vi "modbus-to-real.vi"(8 "error in (no error)":errorcluster, 11 "object in":refnum<class "Pressure-Transducer.lvclass">) -> (0 "error out":errorcluster, 3 "object out":refnum<class "Pressure-Transducer.lvclass">)   [LabVIEW 2021, in "Pressure-Transducer.lvclass"]
doc: "Uses adam formula to convert sensors to real No"
uses:
  Pressure-Transducer.lvclass
panel:
  # "Conversion for 4 to 20mA  and 0 to 10Vdc\ntransducer for the adam 4018+\n\nOutput the 4mA been subtracted."
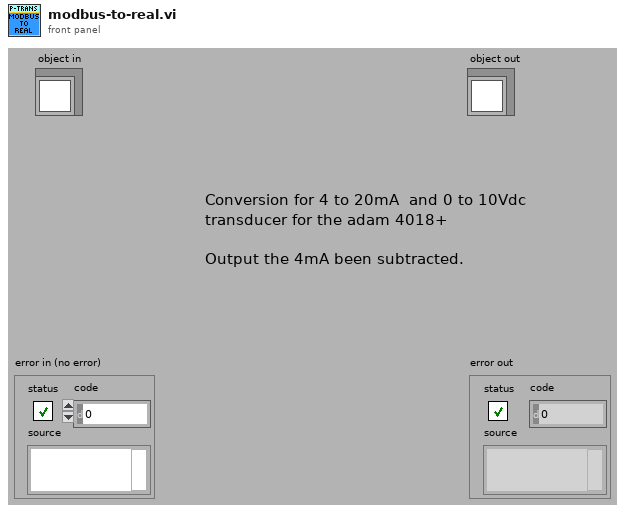
[diagram p1: front panel]
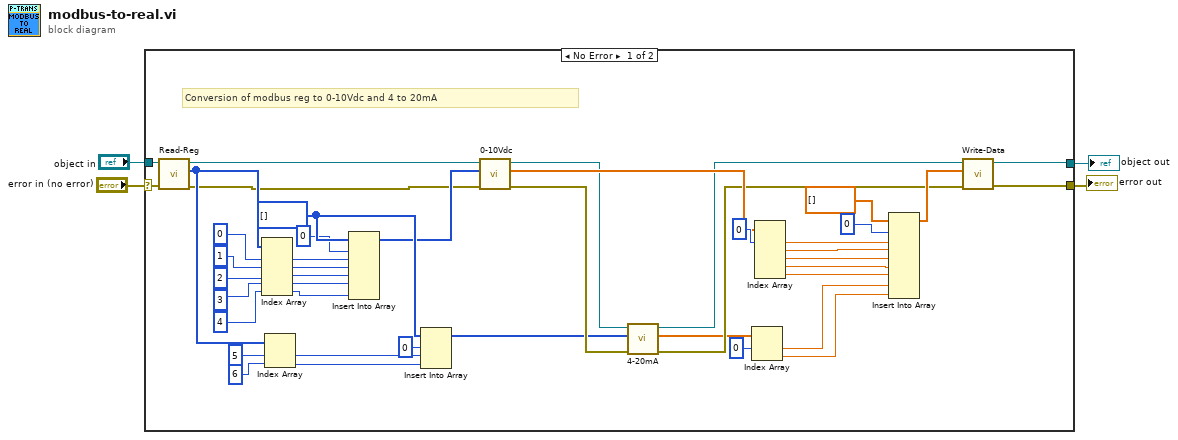
[diagram p0: block diagram]
diagram:
  n1 = case shown="No Error" "error in (no error)" {
    selector: "error in (no error)" -> [w45 w50]
    tunnel: [w47 w50] -> w3
    tunnel: [w48 w49] -> w1
    tunnel: "object in" -> [w46 w49]
    frame No Error {
      w36 = u16[] [] ("array")
      # "Conversion of modbus reg to 0-10Vdc and 4 to 20mA"
      n2 = call-dynamic "Read-Reg.vi"("error in (no error)"=w45, "Type-K-Thermocouple in"=w46) -> ("error out"=w12:errorcluster, "Modbus-Reg"=w39:u16[], "Type-K-Thermocouple out"=w14:refnum<class "Pressure-Transducer.lvclass">)  [unwired: 7 in]
      n3 = Index Array(array=w39, index #1=0 ("index"), index #2=1 ("index"), index #3=2 ("index"), index #4=3 ("index"), index #5=4 ("index")) -> (element #1=w34:u16, element #2=w33:u16, element #3=w32:u16, element #4=w31:u16, element #5=w30:u16)
      n4 = Index Array(array=w39, index #1=5 ("index"), index #2=6 ("index")) -> (element #1=w28:u16, element #2=w27:u16)
      n5 = Insert Into Array(array=w36, index=0, new element #1=w34, new element #2=w33, new element #3=w32, new element #4=w31, new element #5=w30) -> (w13:u16[])
      n6 = Insert Into Array(array=w36, index=0, new element #1=w28, new element #2=w27) -> (w8:u16[])
      n7 = call "0-10Vdc.vi"("error in (no error)"=w12, "Reg Array"=w13, "object in"=w14) -> ("error out"=w9:errorcluster, "0-10Vdc Data"=w11:dbl[], "object out"=w10:refnum<class "Pressure-Transducer.lvclass">)  [unwired: 5 in, 1 out]
      n8 = call "4-20mA.vi"("error in (no error)"=w9, "Reg array"=w8, "object in"=w10) -> ("error out"=w6:errorcluster, "4-20mA Array"=w5:dbl[], "object out"=w7:refnum<class "Pressure-Transducer.lvclass">)  [unwired: 5 in, 1 out]
      n9 = Index Array(array=w5, index #1=0 ("index")) -> (element #1=w17:dbl, element #2=w16:dbl)  [unwired: 1 in]
      n10 = Index Array(array=w11, index #1=0 ("index")) -> (element #1=w22:dbl, element #2=w21:dbl, element #3=w20:dbl, element #4=w19:dbl, element #5=w18:dbl)  [unwired: 4 in]
      n11 = Insert Into Array(array=dbl[] [], index=0, new element #1=w22, new element #2=w21, new element #3=w20, new element #4=w19, new element #5=w18, new element #6=w17, new element #7=w16) -> (w15:dbl[])
      n12 = call-dynamic "Write-Data.vi"("error in (no error)"=w6, "Data"=w15, "Type-K-Thermocouple in"=w7) -> ("error out"=w47:errorcluster, "Type-K-Thermocouple out"=w48:refnum<class "Pressure-Transducer.lvclass">)  [unwired: 7 in]
    }
    frame Error {
    }
  }
  "error out" <- w3
  "object out" <- w1
